vi "Fit.vi"(8 "error in (no error)":errorcluster caption="entrée d'erreur (pas d'erreur)", 10 "y":string[][](array[string]), 11 "MultiLabelBinarizer.lvclass":refnum<class "MultiLabelBinarizer.lvclass">) -> (0 "error out":errorcluster caption="sortie d'erreur", 2 "String Data":string, 3 "MultiLabelBinarizer.lvclass":refnum<class "MultiLabelBinarizer.lvclass">)   [LabVIEW 2020, in "MultiLabelBinarizer.lvclass"]
doc: "Fit the label sets binarizer.\n\nReturns : \n\n- String : OK"
uses:
  MultiLabelBinarizer.lvclass
  MultiLabelBinarizer.lvclass/MultiLabelBinarizer.ctl
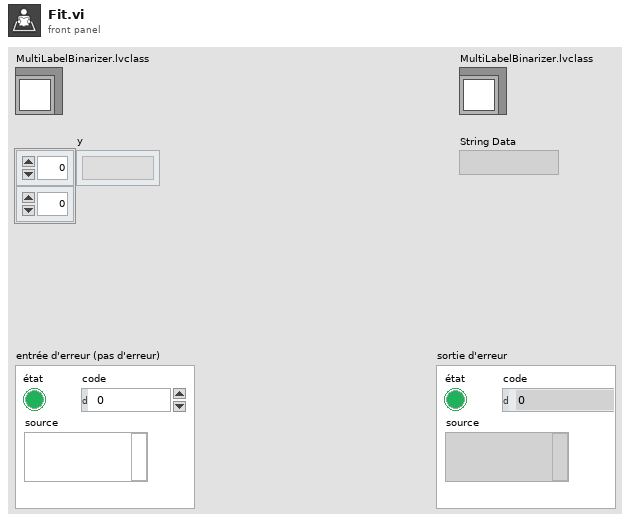
[diagram p1: front panel]
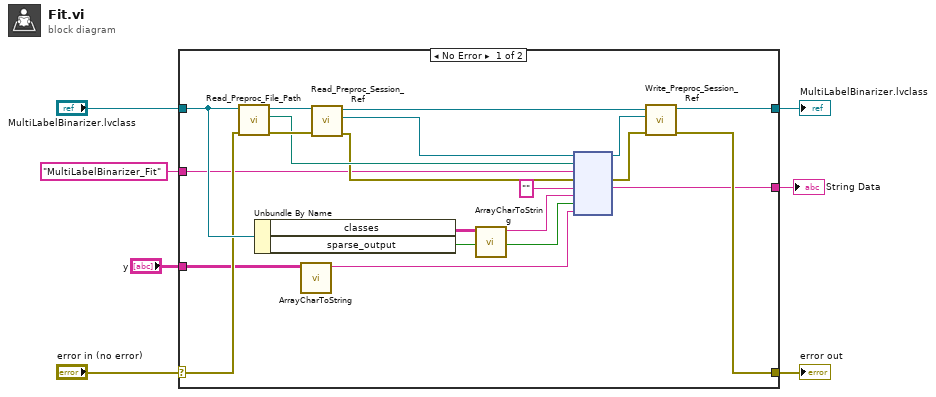
[diagram p0: block diagram]
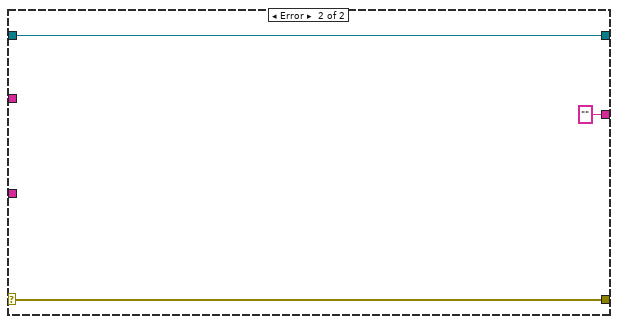
[diagram p2: hidden frame]
diagram:
  n1 = case shown="No Error" "error in (no error)" {
    selector: "error in (no error)" -> [w15 w30]
    tunnel: [w16 w30] -> w6
    tunnel: [w17 w29] -> w4
    tunnel: "MultiLabelBinarizer.lvclass" -> [w18 w29]
    tunnel: "MultiLabelBinarizer_Fit" ("Fonction") -> [w14 _]
    tunnel: [w13 ""] -> w2
    tunnel: "y" -> [w11 _]
    frame No Error {
      n2 = call-dynamic "Read_Preproc_File_Path.vi"("error in (no error)"=w15, "Python in"=w18) -> ("error out"=w26:errorcluster, "File_Path"=w23:path, "Python out"=w27:refnum<class "MultiLabelBinarizer.lvclass">)  [unwired: 7 in]
      n3 = Unbundle By Name(w18) -> ("classes"=w9:string[][], "sparse_output"=w12:bool)
      n4 = call "ArrayCharToString.vi"("TAB"=w11) -> ("Instruction"=w10:string)  [unwired: 10 in]
      n5 = call-dynamic "Read_Preproc_Session_Ref.vi"("error in (no error)"=w26, "Python in"=w27) -> ("error out"=w22:errorcluster, "Session_ref"=w24:refnum<k35>, "Python out"=w25:refnum<class "MultiLabelBinarizer.lvclass">)  [unwired: 7 in]
      n6 = call "ArrayCharToString.vi"("TAB"=w9) -> ("Instruction"=w8:string)  [unwired: 10 in]
      n7 = node(w24, w23, w14, w22, "", w8, w12, w10) -> (w20:refnum<k35>, w21:errorcluster, w13:string)  [unwired: 3 in, 2 out]
      n8 = call-dynamic "Write_Preproc_Session_Ref.vi"("error in (no error)"=w21, "Session_ref"=w20, "Python in"=w25) -> ("error out"=w16:errorcluster, "Python out"=w17:refnum<class "MultiLabelBinarizer.lvclass">)  [unwired: 7 in]
    }
    frame Error {
    }
  }
  "error out" <- w6
  "MultiLabelBinarizer.lvclass" <- w4
  "String Data" <- w2
